vi "Slider Set Limit.vi"(0 "DofType":T3, 5 "LBCB Number":T2, 7 "Value":dbl, 9 "Index":i32, 11 "error in (no error)":errorcluster, 12 "Lower/Upper":T1) -> (15 "error out":errorcluster)   [LabVIEW 2013]
uses:
  Data Access Objects/Limits/DofTypes.ctl
  Data Access Objects/Metadata/LBCB Number.ctl
  Lower Upper Select.ctl
  Data Access Objects/Metadata/Persistant DAO Actions.ctl
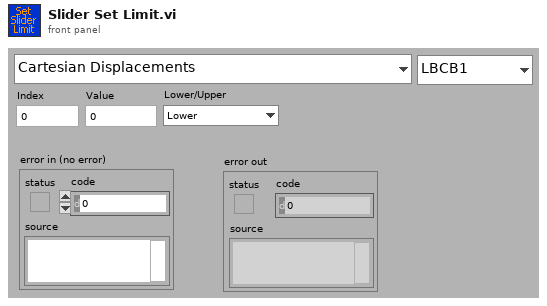
[diagram p1: front panel]
types:
  T1 = typedef "Lower Upper Select.ctl" = enum16{"Lower", "Upper"}
  T2 = typedef "LBCB Number.ctl" = enum16{"LBCB1", "LBCB2"}
  T3 = typedef "DofTypes.ctl" = enum16{"Cartesian Displacements", "Cartesian Forces & Moments", "Actuator Displacements", "Actuator Forces", "Cartesian Increments", "Actuator Increments"}
  T4 = typedef "Persistant DAO Actions.ctl" = enum16{"Init", "Get", "Set", "Load", "Save"}
  T5 = typedef "Cartesian Matrix.ctl" = cluster{"Lower":T6, "Upper":T6}
  T6 = typedef "Cartesian Point.ctl" = cluster{"Dx":dbl, "Dy":dbl, "Dz":dbl, "Rx":dbl, "Ry":dbl, "Rz":dbl}
  T7 = typedef "Limit Matrix.ctl" = dbl[][]
  T8 = typedef "Actuator Point.ctl" = cluster{"X1":dbl, "X2":dbl, "Y1":dbl, "Z1":dbl, "Z2":dbl, "Z3":dbl}
  T9 = typedef "Actuator Matrix.ctl" = cluster{"Lower":T8, "Upper":T8}
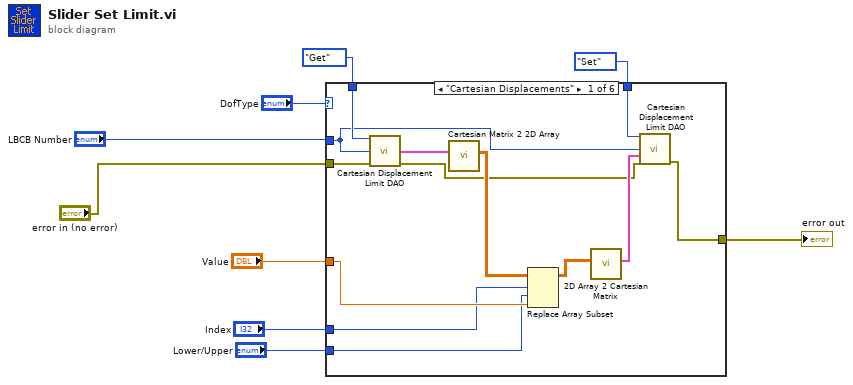
[diagram p0: block diagram]
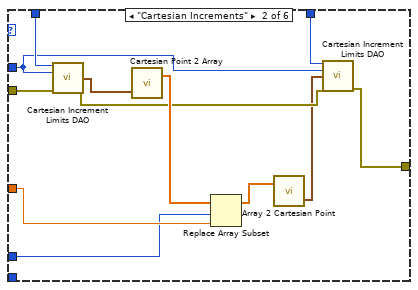
[diagram p2: hidden frame]
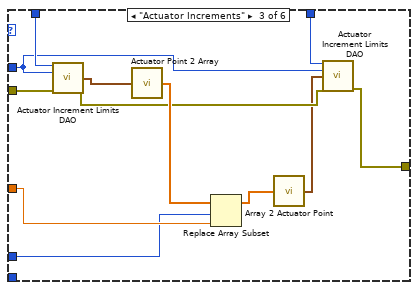
[diagram p3: hidden frame]
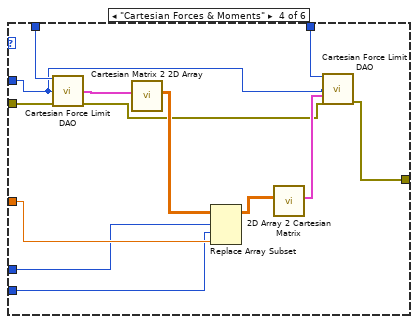
[diagram p4: hidden frame]
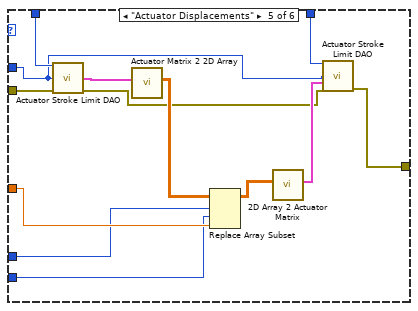
[diagram p5: hidden frame]
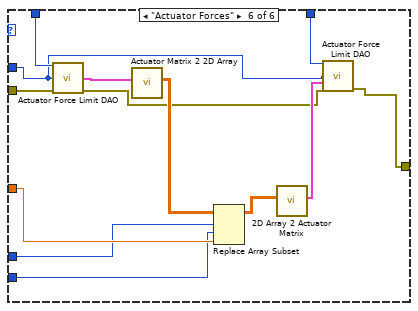
[diagram p6: hidden frame]
diagram:
  n1 = case shown="\"Cartesian Displacements\"" "DofType" {
    tunnel: Persistant_DAO_Actions."Get" ("Cartesian Displacement Limit Actions") -> [w22 w34 w46 w59 w72 w85]
    tunnel: "LBCB Number" -> [w19 w32 w44 w56 w69 w82]
    tunnel: Persistant_DAO_Actions."Set" ("Cartesian Displacement Limit Actions") -> [w20 w33 w45 w57 w70 w83]
    tunnel: "Lower/Upper" -> [w11 _ _ w47 w60 w73]
    tunnel: "Index" -> [w10 w25 w37 w48 w61 w74]
    tunnel: "Value" -> [w17 w30 w42 w54 w67 w80]
    tunnel: "error in (no error)" -> [w14 w28 w40 w51 w64 w77]
    tunnel: [w12 w26 w38 w49 w62 w75] -> w1
    frame "Cartesian Displacements" {
      n2 = call "Cartesian Displacement Limit DAO.vi"("Cartesian Displacement Limit Actions"=w22, "ID"=w19, "error in (no error)"=w14) -> ("Cartesian Displacement Out"=w21:T5, "error out"=w13:errorcluster)  [unwired: 10 in, 1 out]
      n3 = call "Cartesian Matrix 2 2D Array.vi"("Matrix In"=w21) -> ("Matrix Out"=w18:T7)  [unwired: 10 in]
      n4 = Replace Array Subset(array=w18, new element=w17, index (row)=w10, index (col)=w11) -> (w16:T7)
      n5 = call "2D Array 2 Cartesian Matrix.vi"("Matrix In"=w16) -> ("Matrix Out"=w15:T5)  [unwired: 10 in]
      n6 = call "Cartesian Displacement Limit DAO.vi"("Cartesian Displacement Limit Actions"=w20, "ID"=w19, "Cartesian Displacement In"=w15, "error in (no error)"=w13) -> ("error out"=w12:errorcluster)  [unwired: 9 in, 2 out]
    }
    frame "Cartesian Increments" {
      n7 = call "Cartesian Increment Limits DAO.vi"("Actions"=w34, "LBCB Number"=w32, "error in (no error)"=w28) -> ("Inc Limits Out"=w24:T6, "error out"=w27:errorcluster)  [unwired: 10 in, 1 out]
      n8 = call "Cartesian Point 2 Array.vi"("Cart Disp"=w24) -> ("Array"=w31:dbl[])  [unwired: 2 in]
      n9 = Replace Array Subset(array=w31, new element=w30, index=w25) -> (w29:dbl[])
      n10 = call "Array 2 Cartesian Point.vi"("Array"=w29) -> ("Cart Disp"=w23:T6)  [unwired: 2 in]
      n11 = call "Cartesian Increment Limits DAO.vi"("Actions"=w33, "LBCB Number"=w32, "Inc Limits In"=w23, "error in (no error)"=w27) -> ("error out"=w26:errorcluster)  [unwired: 9 in, 2 out]
    }
    frame "Actuator Increments" {
      n12 = call "Actuator Increment Limits DAO.vi"("Actions"=w46, "LBCB Number"=w44, "error in (no error)"=w40) -> ("Inc Limits Out"=w36:T8, "error out"=w39:errorcluster)  [unwired: 10 in, 1 out]
      n13 = call "Actuator Point 2 Array.vi"("Actuator Point"=w36) -> ("Array"=w43:dbl[])
      n14 = Replace Array Subset(array=w43, new element=w42, index=w37) -> (w41:dbl[])
      n15 = call "Array 2 Actuator Point.vi"("Array"=w41) -> ("Actuator Point"=w35:T8)
      n16 = call "Actuator Increment Limits DAO.vi"("Actions"=w45, "LBCB Number"=w44, "Inc Limits In"=w35, "error in (no error)"=w39) -> ("error out"=w38:errorcluster)  [unwired: 9 in, 2 out]
    }
    frame "Cartesian Forces & Moments" {
      n17 = call "Cartesian Force Limit DAO.vi"("Cartesian Force Limit Actions"=w59, "ID"=w56, "error in (no error)"=w51) -> ("Cartesian Force Limit Out"=w58:T5, "error out"=w50:errorcluster)  [unwired: 10 in, 1 out]
      n18 = call "Cartesian Matrix 2 2D Array.vi"("Matrix In"=w58) -> ("Matrix Out"=w55:T7)  [unwired: 10 in]
      n19 = Replace Array Subset(array=w55, new element=w54, index (row)=w48, index (col)=w47) -> (w53:T7)
      n20 = call "2D Array 2 Cartesian Matrix.vi"("Matrix In"=w53) -> ("Matrix Out"=w52:T5)  [unwired: 10 in]
      n21 = call "Cartesian Force Limit DAO.vi"("Cartesian Force Limit Actions"=w57, "ID"=w56, "Cartesian Force Limit In"=w52, "error in (no error)"=w50) -> ("error out"=w49:errorcluster)  [unwired: 9 in, 2 out]
    }
    frame "Actuator Displacements" {
      n22 = call "Actuator Stroke Limit DAO.vi"("Actuator Stroke Limit Actions"=w72, "ID"=w69, "error in (no error)"=w64) -> ("Actuator Stroke Limits Out"=w71:T9, "error out"=w63:errorcluster)  [unwired: 10 in, 1 out]
      n23 = call "Actuator Matrix 2 2D Array.vi"("Matrix In"=w71) -> ("Matrix Out"=w68:T7)  [unwired: 10 in]
      n24 = Replace Array Subset(array=w68, new element=w67, index (row)=w61, index (col)=w60) -> (w66:T7)
      n25 = call "2D Array 2 Actuator Matrix.vi"("Matrix In"=w66) -> ("Matrix Out"=w65:T9)  [unwired: 10 in]
      n26 = call "Actuator Stroke Limit DAO.vi"("Actuator Stroke Limit Actions"=w70, "ID"=w69, "Actuator Stroke Limits In"=w65, "error in (no error)"=w63) -> ("error out"=w62:errorcluster)  [unwired: 9 in, 2 out]
    }
    frame "Actuator Forces" {
      n27 = call "Actuator Force Limit DAO.vi"("Actuator Force Limit Actions"=w85, "ID"=w82, "error in (no error)"=w77) -> ("Actuator Force Limits Out"=w84:T9, "error out"=w76:errorcluster)  [unwired: 10 in, 1 out]
      n28 = call "Actuator Matrix 2 2D Array.vi"("Matrix In"=w84) -> ("Matrix Out"=w81:T7)  [unwired: 10 in]
      n29 = Replace Array Subset(array=w81, new element=w80, index (row)=w74, index (col)=w73) -> (w79:T7)
      n30 = call "2D Array 2 Actuator Matrix.vi"("Matrix In"=w79) -> ("Matrix Out"=w78:T9)  [unwired: 10 in]
      n31 = call "Actuator Force Limit DAO.vi"("Actuator Force Limit Actions"=w83, "ID"=w82, "Actuator Force Limits  Input"=w78, "error in (no error)"=w76) -> ("error out"=w75:errorcluster)  [unwired: 9 in, 2 out]
    }
  }
  "error out" <- w1
